vi "Gif.LogicalScreenDescriptor.vi"(0 "data":string, 9 "offset":i32, 11 "error in (no error)":errorcluster) -> (4 "data out":string, 6 "Logical Screen Descriptor":T1, 10 "offset out":i32, 15 "error out":errorcluster)   [LabVIEW 2019]
doc: "This vi reads the Logical Screen Description. The length of the Logical Screen Descriptor is seven bytes. The detailed description can be found in chapter x in \"http://www.w3.org/Graphics/GIF/spec-gif89a.txt\""
uses:
  Gif.LogicalScreenDescriptior.ctl
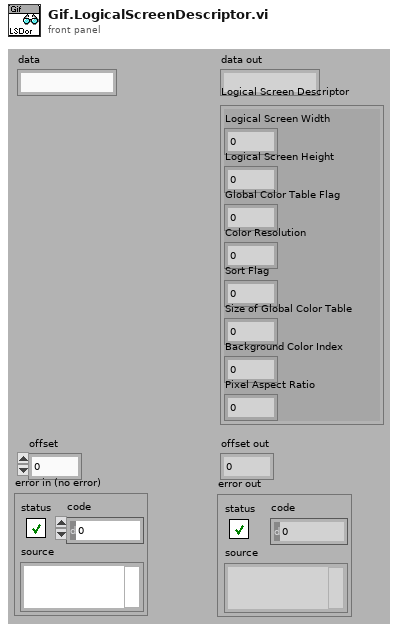
[diagram p1: front panel]
types:
  T1 = typedef "Gif.LogicalScreenDescriptior.ctl" = cluster{"Logical Screen Width":u16, "Logical Screen Height":u16, "Global Color Table Flag":u8, "Color Resolution":u8, "Sort Flag":u8, "Size of Global Color Table":u8, "Background Color Index":u8, "Pixel Aspect Ratio":u8}
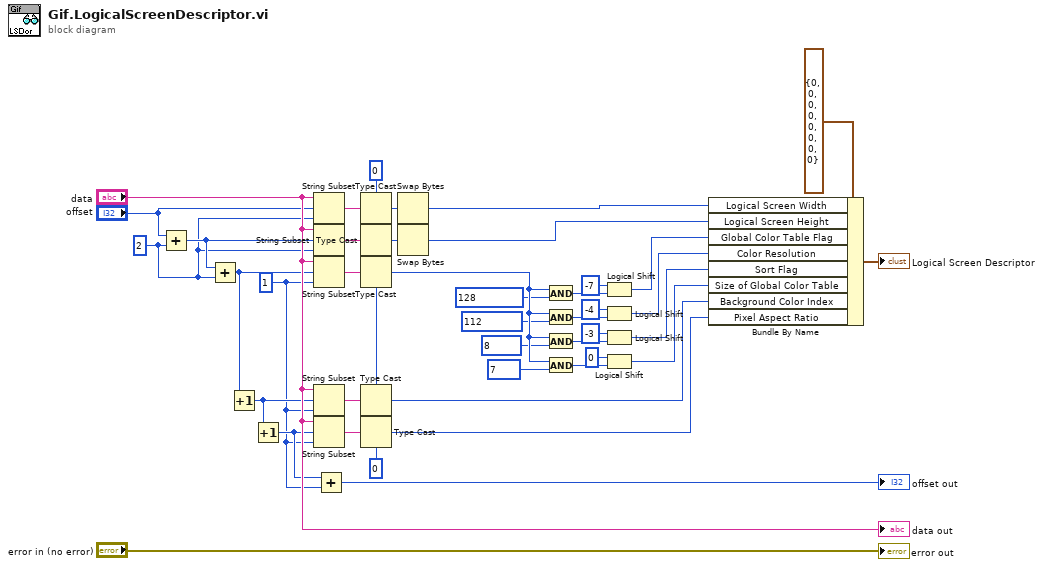
[diagram p0: block diagram]
diagram:
  w28 = u8 0 ("length (rest)")
  w33 = u16 0 ("length (rest)")
  w25 = 1 ("length (rest)")
  w24 = 2 ("length (rest)")
  n1 = Add(x="offset", y=w24) -> (x+y=w39:i32)
  n2 = Add(x=w39, y=w24) -> (x+y=w38:i32)
  n3 = Increment(x=w38) -> (x+1=w37:i32)
  n4 = Increment(x=w37) -> (x+1=w26:i32)
  n5 = String Subset(string="data", offset (0)="offset", length (rest)=w24) -> (substring=w36:string)
  n6 = String Subset(string="data", offset (0)=w39, length (rest)=w24) -> (substring=w34:string)
  n7 = String Subset(string="data", offset (0)=w38, length (rest)=w25) -> (substring=w29:string)
  n8 = String Subset(string="data", offset (0)=w37, length (rest)=w25) -> (substring=w31:string)
  n9 = String Subset(string="data", offset (0)=w26, length (rest)=w25) -> (substring=w30:string)
  n10 = Add(x=w26, y=w25) -> (x+y=→"offset out":i32)
  n11 = Type Cast(type=w33, x=w36) -> (*(type *) &x=w35:u16)
  n12 = Type Cast(type=w33, x=w34) -> (*(type *) &x=w32:u16)
  n13 = Type Cast(type=w28, x=w29) -> (*(type *) &x=w27:u8)
  n14 = Type Cast(type=w28, x=w31) -> (*(type *) &x=w17:u8)
  n15 = Type Cast(type=w28, x=w30) -> (*(type *) &x=w16:u8)
  n16 = Swap Bytes(anything=w35) -> (byte swapped=w22:u16)
  n17 = Swap Bytes(anything=w32) -> (byte swapped=w21:u16)
  n18 = And(x=w27, y=u8 128) -> (x .and. y?=w2:u8)
  n19 = And(x=w27, y=u8 112) -> (x .and. y?=w8:u8)
  n20 = And(x=w27, y=u8 8) -> (x .and. y?=w7:u8)
  n21 = And(x=w27, y=u8 7) -> (x .and. y?=w6:u8)
  n22 = Logical Shift(y=-7, x=w2) -> (x << y=w15:u8)
  n23 = Logical Shift(y=-4, x=w8) -> (x << y=w20:u8)
  n24 = Logical Shift(y=-3, x=w7) -> (x << y=w19:u8)
  n25 = Logical Shift(y=0, x=w6) -> (x << y=w18:u8)
  n26 = Bundle By Name(cluster=T1 {"Logical Screen Width"=0, "Logical Screen Height"=0, "Global Color Table Flag"=0, "Color Resolution"=0, "Sort Flag"=0, "Size of Global Color Table"=0, "Background Color Index"=0, "Pixel Aspect Ratio"=0} ("Logical Screen Description"), "Logical Screen Width"=w22, "Logical Screen Height"=w21, "Global Color Table Flag"=w15, "Color Resolution"=w20, "Sort Flag"=w19, "Size of Global Color Table"=w18, "Background Color Index"=w17, "Pixel Aspect Ratio"=w16) -> (→"Logical Screen Descriptor":T1)
  "data out" <- "data"
  "error out" <- "error in (no error)"
